vi "Configuration.vi"(8 "error in (no error)":errorcluster) -> (0 "error out":errorcluster, 3 "Electrical Test Only status":bool)   [LabVIEW 2015]
uses:
  C:/C-BOX_DoIP/Utilities/dotNET/C-BOX_DoIP/INIFileParser.dll
  C-BOX_DoIP/Utilities/dotNET/C-BOX_DoIP/INIFileParser.dll
  C:/C-BOX_DoIP/Utilities/dotNET/C-BOX_DoIP/C_Box.NET_Utilities.dll
  C-BOX_DoIP/Utilities/dotNET/C-BOX_DoIP/C_Box.NET_Utilities.dll
panel:
  in  "Cancel Button":bool
  in  "Save Button":bool
  in  "Tab Control":enum32{"Parametros de estación"}(tab)
  in  "Electrical Test Checkbox":bool caption="Solo prueba eléctrica:"
  in  "FAZIT tester id":string caption="Tester ID FAZIT:"
  in  "MAC Address password":string caption="Contraseña MAC Address:"
  in  "MAC Address user":string caption="Usuario MAC Address:"
  in  "DB MAC Address":string caption="Base de datos MAC Address:"
  in  "Server MAC Address":string caption="Servidor MAC Address:"
  in  "Station ID":string caption="ID de estación:"
  in  "Plant number":string caption="Plant number:"
  in  "Producer code":string caption="Producer code:"
  in  "Nest data folder":path caption="Directorio información de nidos:"
  in  "GNSS scenario file":string caption="Archivo escenario GNSS:"
  in  "Instruments file":path caption="Archivo de instrumentos:"
  in  "Variants file":path caption="Archivo de variantes:"
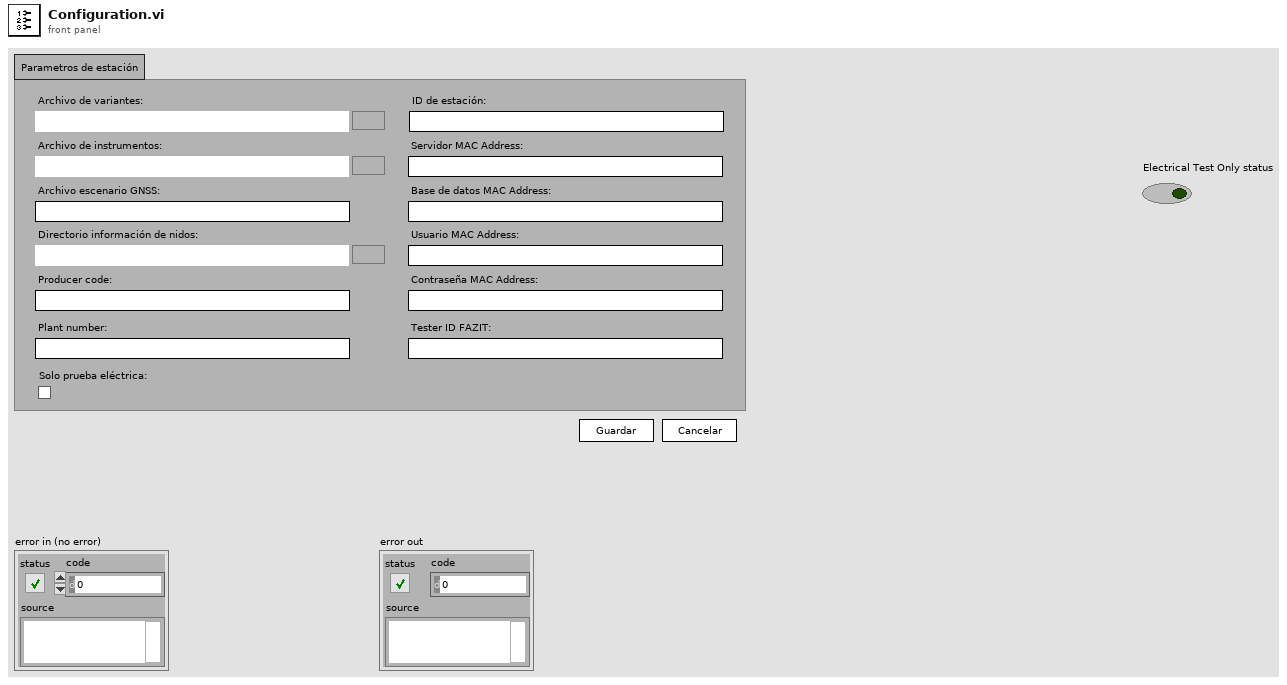
[diagram p1: front panel]
types:
  T1 = enum16{"Init", "Read system settings", "Event handler", "Write system settings", "Exit"}
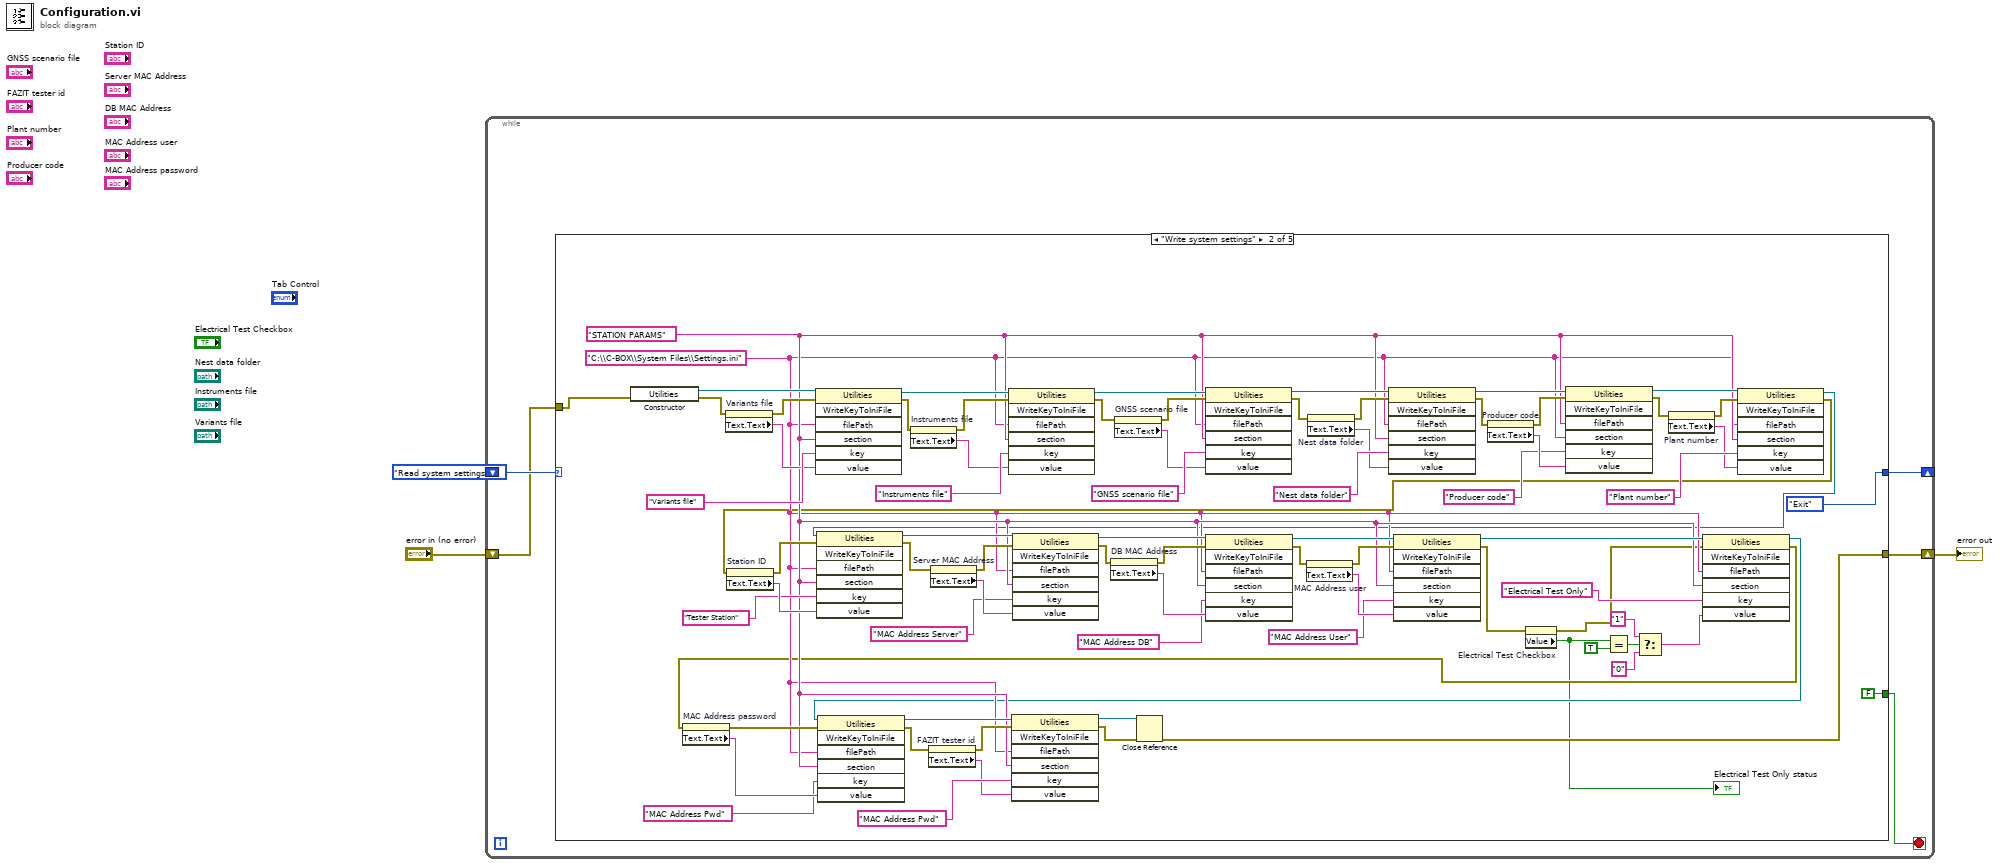
[diagram p0: block diagram]
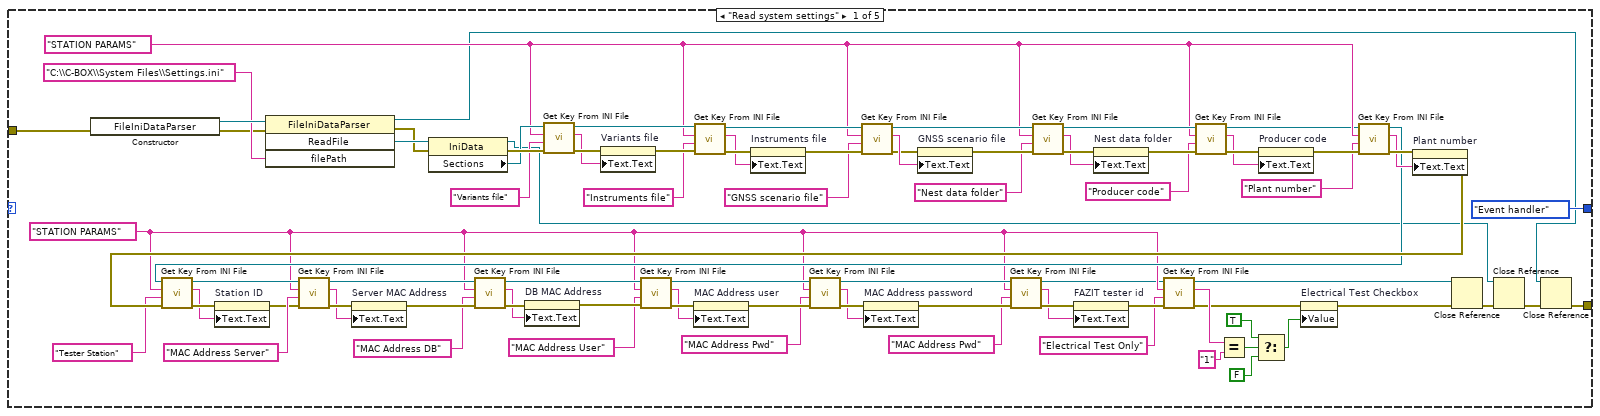
[diagram p2: hidden frame]
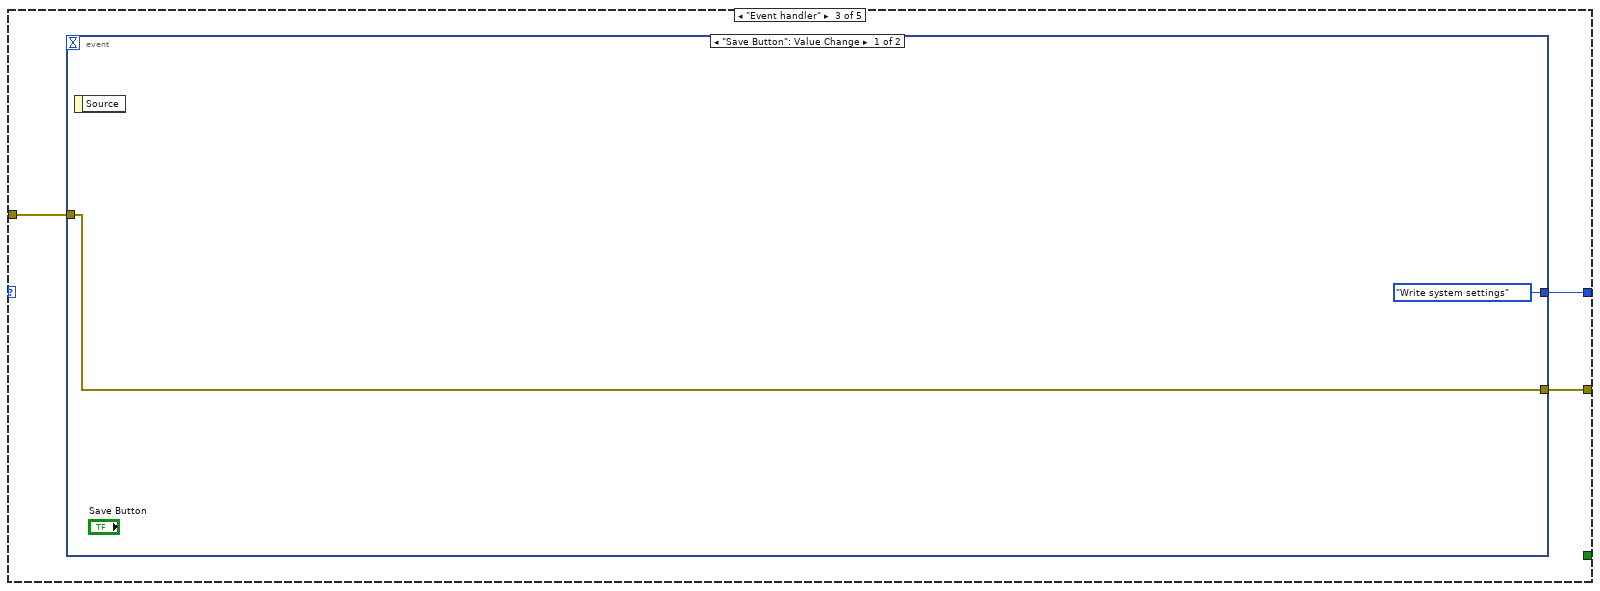
[diagram p3: hidden frame]
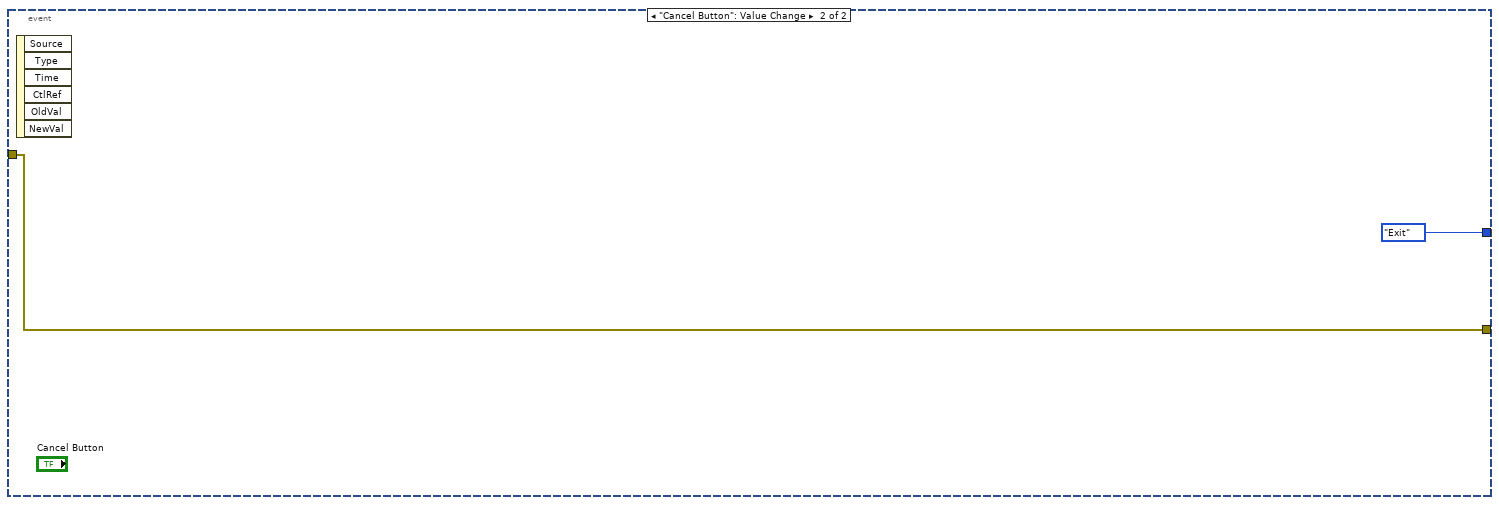
[diagram p4: hidden frame]
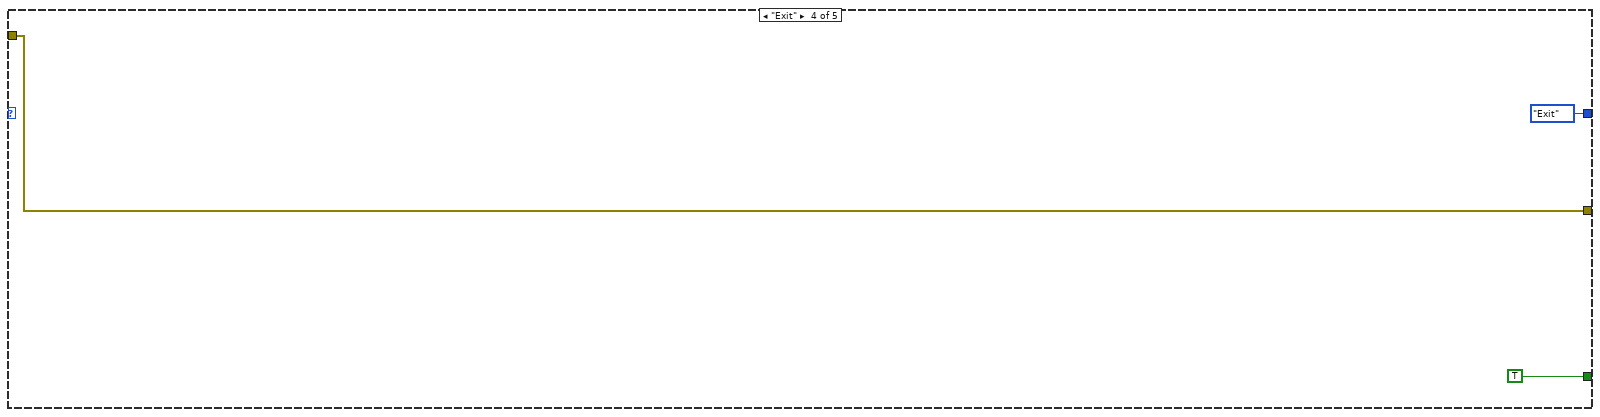
[diagram p5: hidden frame]
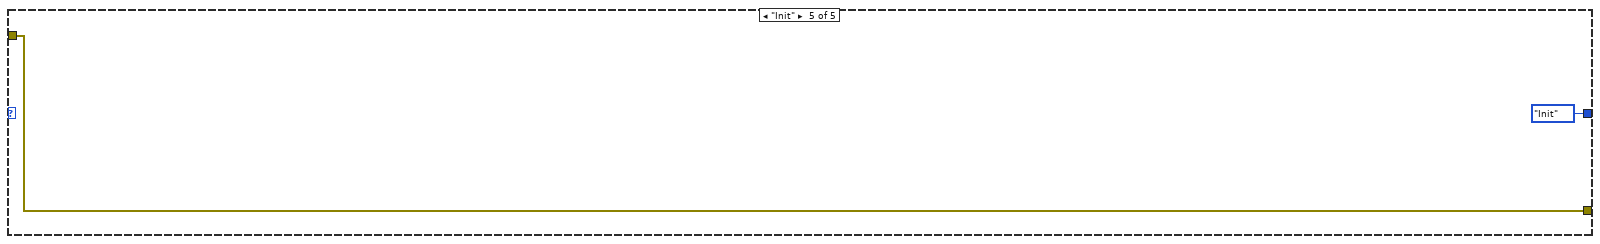
[diagram p6: hidden frame]
diagram:
  n1 = while {
    shift-right: [w6] -> w1
    shift-left: "error in (no error)" -> [w7]
    shift-right: [w5] -> _
    shift-left: T1."Read system settings" -> [w8]
    stop <- w4 stop-if-true
    n2 = case shown="\"Write system settings\"" w8 {
      tunnel: w7 -> [w79 w95 w174 w180 w183]
      tunnel: [w12 w100 w173 w180 w183] -> w6
      tunnel: [T1."Event handler" T1."Exit" w175 T1."Exit" T1."Init"] -> w5
      tunnel: [_ FALSE _ TRUE _] -> w4
      frame "Read system settings" {
        w26 = "STATION PARAMS" ("sectionName")
        w62 = "STATION PARAMS" ("sectionName")
        n3 = constructor class="FileIniDataParser"(error in=w79) -> (reference out=w94:refnum<k24>, error out=w89:errorcluster)  [unwired: 2 in, 1 out]
        n4 = invoke class="FileIniDataParser" method="ReadFile"(reference=w94, error in=w89, "filePath"="C:\\C-BOX\\System Files\\Settings.ini") -> (reference out=w9:refnum<k24>, error out=w90:errorcluster, "ReadFile"=w92:refnum<k24>)  [unwired: 1 in, 1 out]
        n5 = property class="IniData"(reference=w92, error in=w90) -> (reference out=w10:refnum<k24>, error out=w91:errorcluster, "Sections"=w88:refnum<k24>)
        n6 = call "Get Key From INI File.vi"("error in (no error)"=w91, "keyName"="Variants file", "sectionName"=w62, "Sections in"=w88) -> ("error out"=w87:errorcluster, "keyValue"=w84:string, "Sections out"=w83:refnum<k24>)  [unwired: 5 in]
        n7 = property on="Variants file" class="Path"(error in=w87, "Text.Text"=w84) -> (error out=w86:errorcluster)  [unwired: 1 in, 1 out]
        n8 = call "Get Key From INI File.vi"("error in (no error)"=w86, "keyName"="Instruments file", "sectionName"=w62, "Sections in"=w83) -> ("error out"=w81:errorcluster, "keyValue"=w80:string, "Sections out"=w76:refnum<k24>)  [unwired: 5 in]
        n9 = property on="Instruments file" class="Path"(error in=w81, "Text.Text"=w80) -> (error out=w78:errorcluster)  [unwired: 1 in, 1 out]
        n10 = call "Get Key From INI File.vi"("error in (no error)"=w78, "keyName"="GNSS scenario file", "sectionName"=w62, "Sections in"=w76) -> ("error out"=w74:errorcluster, "keyValue"=w75:string, "Sections out"=w72:refnum<k24>)  [unwired: 5 in]
        n11 = property on="GNSS scenario file" class="Str"(error in=w74, "Text.Text"=w75) -> (error out=w73:errorcluster)  [unwired: 1 in, 1 out]
        n12 = call "Get Key From INI File.vi"("error in (no error)"=w73, "keyName"="Nest data folder", "sectionName"=w62, "Sections in"=w72) -> ("error out"=w70:errorcluster, "keyValue"=w69:string, "Sections out"=w67:refnum<k24>)  [unwired: 5 in]
        n13 = property on="Nest data folder" class="Path"(error in=w70, "Text.Text"=w69) -> (error out=w68:errorcluster)  [unwired: 1 in, 1 out]
        n14 = call "Get Key From INI File.vi"("error in (no error)"=w68, "keyName"="Producer code", "sectionName"=w62, "Sections in"=w67) -> ("error out"=w65:errorcluster, "keyValue"=w64:string, "Sections out"=w61:refnum<k24>)  [unwired: 5 in]
        n15 = property on="Producer code" class="Str"(error in=w65, "Text.Text"=w64) -> (error out=w63:errorcluster)  [unwired: 1 in, 1 out]
        n16 = call "Get Key From INI File.vi"("error in (no error)"=w63, "keyName"="Plant number", "sectionName"=w62, "Sections in"=w61) -> ("error out"=w59:errorcluster, "keyValue"=w58:string, "Sections out"=w56:refnum<k24>)  [unwired: 5 in]
        n17 = property on="Plant number" class="Str"(error in=w59, "Text.Text"=w58) -> (error out=w57:errorcluster)  [unwired: 1 in, 1 out]
        n18 = call "Get Key From INI File.vi"("error in (no error)"=w57, "keyName"="Tester Station", "sectionName"=w26, "Sections in"=w56) -> ("error out"=w52:errorcluster, "keyValue"=w51:string, "Sections out"=w54:refnum<k24>)  [unwired: 5 in]
        n19 = property on="Station ID" class="Str"(error in=w52, "Text.Text"=w51) -> (error out=w50:errorcluster)  [unwired: 1 in, 1 out]
        n20 = call "Get Key From INI File.vi"("error in (no error)"=w50, "keyName"="MAC Address Server", "sectionName"=w26, "Sections in"=w54) -> ("error out"=w49:errorcluster, "keyValue"=w48:string, "Sections out"=w46:refnum<k24>)  [unwired: 5 in]
        n21 = property on="Server MAC Address" class="Str"(error in=w49, "Text.Text"=w48) -> (error out=w47:errorcluster)  [unwired: 1 in, 1 out]
        n22 = call "Get Key From INI File.vi"("error in (no error)"=w47, "keyName"="MAC Address DB", "sectionName"=w26, "Sections in"=w46) -> ("error out"=w44:errorcluster, "keyValue"=w43:string, "Sections out"=w42:refnum<k24>)  [unwired: 5 in]
        n23 = property on="DB MAC Address" class="Str"(error in=w44, "Text.Text"=w43) -> (error out=w41:errorcluster)  [unwired: 1 in, 1 out]
        n24 = call "Get Key From INI File.vi"("error in (no error)"=w41, "keyName"="MAC Address User", "sectionName"=w26, "Sections in"=w42) -> ("error out"=w39:errorcluster, "keyValue"=w38:string, "Sections out"=w36:refnum<k24>)  [unwired: 5 in]
        n25 = property on="MAC Address user" class="Str"(error in=w39, "Text.Text"=w38) -> (error out=w37:errorcluster)  [unwired: 1 in, 1 out]
        n26 = call "Get Key From INI File.vi"("error in (no error)"=w37, "keyName"="MAC Address Pwd", "sectionName"=w26, "Sections in"=w36) -> ("error out"=w34:errorcluster, "keyValue"=w33:string, "Sections out"=w31:refnum<k24>)  [unwired: 5 in]
        n27 = property on="MAC Address password" class="Str"(error in=w34, "Text.Text"=w33) -> (error out=w32:errorcluster)  [unwired: 1 in, 1 out]
        n28 = call "Get Key From INI File.vi"("error in (no error)"=w32, "keyName"="MAC Address Pwd", "sectionName"=w26, "Sections in"=w31) -> ("error out"=w29:errorcluster, "keyValue"=w28:string, "Sections out"=w25:refnum<k24>)  [unwired: 5 in]
        n29 = property on="FAZIT tester id" class="Str"(error in=w29, "Text.Text"=w28) -> (error out=w27:errorcluster)  [unwired: 1 in, 1 out]
        n30 = call "Get Key From INI File.vi"("error in (no error)"=w27, "keyName"="Electrical Test Only", "sectionName"=w26, "Sections in"=w25) -> ("error out"=w18:errorcluster, "keyValue"=w23:string, "Sections out"=w16:refnum<k24>)  [unwired: 5 in]
        n31 = Equal?(x=w23, y="1") -> (x = y?=w24:bool)
        n32 = Select(t=TRUE, s=w24, f=FALSE) -> (s? t:f=w21:bool)
        n33 = property on="Electrical Test Checkbox" class="Bool (strict)"(error in=w18, "Value"=w21) -> (error out=w17:errorcluster)  [unwired: 1 in, 1 out]
        n34 = Close Reference(reference=w16, error in (no error)=w17) -> (error out=w13:errorcluster)
        n35 = Close Reference(reference=w10, error in (no error)=w13) -> (error out=w11:errorcluster)
        n36 = Close Reference(reference=w9, error in (no error)=w11) -> (error out=w12:errorcluster)
      }
      frame "Write system settings" {
        w106 = "STATION PARAMS" ("sectionName")
        w105 = "C:\\C-BOX\\System Files\\Settings.ini" ("filePath")
        n37 = constructor class="Utilities"(error in=w95) -> (reference out=w166:refnum<k24>, error out=w164:errorcluster)  [unwired: 2 in, 1 out]
        n38 = property on="Variants file" class="Path"(error in=w164) -> (error out=w163:errorcluster, "Text.Text"=w162:string)  [unwired: 1 in, 1 out]
        n39 = invoke class="Utilities" method="WriteKeyToIniFile"(reference=w166, error in=w163, "filePath"=w105, "section"=w106, "key"="Variants file" ("keyName"), "value"=w162) -> (reference out=w161:refnum<k24>, error out=w159:errorcluster)  [unwired: 1 in, 5 out]
        n40 = property on="Instruments file" class="Path"(error in=w159) -> (error out=w158:errorcluster, "Text.Text"=w157:string)  [unwired: 1 in, 1 out]
        n41 = invoke class="Utilities" method="WriteKeyToIniFile"(reference=w161, error in=w158, "filePath"=w105, "section"=w106, "key"="Instruments file" ("keyName"), "value"=w157) -> (reference out=w156:refnum<k24>, error out=w155:errorcluster)  [unwired: 1 in, 5 out]
        n42 = property on="GNSS scenario file" class="Str"(error in=w155) -> (error out=w154:errorcluster, "Text.Text"=w152:string)  [unwired: 1 in, 1 out]
        n43 = invoke class="Utilities" method="WriteKeyToIniFile"(reference=w156, error in=w154, "filePath"=w105, "section"=w106, "key"="GNSS scenario file" ("keyName"), "value"=w152) -> (reference out=w149:refnum<k24>, error out=w151:errorcluster)  [unwired: 1 in, 5 out]
        n44 = property on="Nest data folder" class="Path"(error in=w151) -> (error out=w150:errorcluster, "Text.Text"=w147:string)  [unwired: 1 in, 1 out]
        n45 = invoke class="Utilities" method="WriteKeyToIniFile"(reference=w149, error in=w150, "filePath"=w105, "section"=w106, "key"="Nest data folder" ("keyName"), "value"=w147) -> (reference out=w146:refnum<k24>, error out=w145:errorcluster)  [unwired: 1 in, 5 out]
        n46 = property on="Producer code" class="Str"(error in=w145) -> (error out=w144:errorcluster, "Text.Text"=w143:string)  [unwired: 1 in, 1 out]
        n47 = invoke class="Utilities" method="WriteKeyToIniFile"(reference=w146, error in=w144, "filePath"=w106, "section"=w105, "key"="Producer code" ("keyName"), "value"=w143) -> (reference out=w140:refnum<k24>, error out=w141:errorcluster)  [unwired: 1 in, 5 out]
        n48 = property on="Plant number" class="Str"(error in=w141) -> (error out=w139:errorcluster, "Text.Text"=w137:string)  [unwired: 1 in, 1 out]
        n49 = invoke class="Utilities" method="WriteKeyToIniFile"(reference=w140, error in=w139, "filePath"=w105, "section"=w106, "key"="Plant number" ("keyName"), "value"=w137) -> (reference out=w98:refnum<k24>, error out=w99:errorcluster)  [unwired: 1 in, 5 out]
        n50 = property on="Station ID" class="Str"(error in=w99) -> (error out=w136:errorcluster, "Text.Text"=w135:string)  [unwired: 1 in, 1 out]
        n51 = invoke class="Utilities" method="WriteKeyToIniFile"(reference=w98, error in=w136, "filePath"=w105, "section"=w106, "key"="Tester Station" ("keyName"), "value"=w135) -> (reference out=w131:refnum<k24>, error out=w133:errorcluster)  [unwired: 1 in, 5 out]
        n52 = property on="Server MAC Address" class="Str"(error in=w133) -> (error out=w132:errorcluster, "Text.Text"=w130:string)  [unwired: 1 in, 1 out]
        n53 = invoke class="Utilities" method="WriteKeyToIniFile"(reference=w131, error in=w132, "filePath"=w105, "section"=w106, "key"="MAC Address Server" ("keyName"), "value"=w130) -> (reference out=w128:refnum<k24>, error out=w127:errorcluster)  [unwired: 1 in, 5 out]
        n54 = property on="DB MAC Address" class="Str"(error in=w127) -> (error out=w126:errorcluster, "Text.Text"=w125:string)  [unwired: 1 in, 1 out]
        n55 = invoke class="Utilities" method="WriteKeyToIniFile"(reference=w128, error in=w126, "filePath"=w105, "section"=w106, "key"="MAC Address DB" ("keyName"), "value"=w125) -> (reference out=w123:refnum<k24>, error out=w122:errorcluster)  [unwired: 1 in, 5 out]
        n56 = property on="MAC Address user" class="Str"(error in=w122) -> (error out=w121:errorcluster, "Text.Text"=w120:string)  [unwired: 1 in, 1 out]
        n57 = invoke class="Utilities" method="WriteKeyToIniFile"(reference=w123, error in=w121, "filePath"=w105, "section"=w106, "key"="MAC Address User" ("keyName"), "value"=w120) -> (reference out=w118:refnum<k24>, error out=w117:errorcluster)  [unwired: 1 in, 5 out]
        n58 = property on="Electrical Test Checkbox" class="Bool (strict)"(error in=w117) -> (error out=w104:errorcluster, "Value"=w96:bool)  [unwired: 1 in, 1 out]
        "Electrical Test Only status" <- w96
        n59 = Equal?(x=w96, y=TRUE) -> (x = y?=w172:bool)
        n60 = Select(t="1", s=w172, f="0") -> (s? t:f=w116:string)
        n61 = invoke class="Utilities" method="WriteKeyToIniFile"(reference=w118, error in=w104, "filePath"=w105, "section"=w106, "key"="Electrical Test Only" ("keyName"), "value"=w116) -> (reference out=w97:refnum<k24>, error out=w103:errorcluster)  [unwired: 1 in, 5 out]
        n62 = property on="MAC Address password" class="Str"(error in=w103) -> (error out=w114:errorcluster, "Text.Text"=w113:string)  [unwired: 1 in, 1 out]
        n63 = invoke class="Utilities" method="WriteKeyToIniFile"(reference=w97, error in=w114, "filePath"=w105, "section"=w106, "key"="MAC Address Pwd" ("keyName"), "value"=w113) -> (reference out=w109:refnum<k24>, error out=w111:errorcluster)  [unwired: 1 in, 5 out]
        n64 = property on="FAZIT tester id" class="Str"(error in=w111) -> (error out=w110:errorcluster, "Text.Text"=w107:string)  [unwired: 1 in, 1 out]
        n65 = invoke class="Utilities" method="WriteKeyToIniFile"(reference=w109, error in=w110, "filePath"=w105, "section"=w106, "key"="MAC Address Pwd" ("keyName"), "value"=w107) -> (reference out=w102:refnum<k24>, error out=w101:errorcluster)  [unwired: 1 in, 5 out]
        n66 = Close Reference(reference=w102, error in (no error)=w101) -> (error out=w100:errorcluster)
      }
      frame "Event handler" {
        n67 = event shown="[0] \"Save Button\": Value Change" {
          selector: _ -> [_ _]
          dyn-events: _ -> [_ _]
          timeout: _ -> [_ _]
          tunnel: [T1."Write system settings" T1."Exit"] -> w175
          tunnel: w174 -> [w176 w178]
          tunnel: [w176 w178] -> w173
          event "Save Button": Value Change {
            n68 = event-data() -> ()  [unwired: 1 in, 1 out]
          }
          event "Cancel Button": Value Change {
            n69 = event-data() -> ()  [unwired: 1 in, 6 out]
          }
        }
      }
      frame "Exit" {
      }
      frame "Init" {
      }
    }
  }
  "error out" <- w1
